vi "Main.vi"(10 "Game Settings":T1={"Control Device"=enum."Mouse", "Players Number"=4, "Score Limit"=3, "Difficulty"=1.0, "FPS"=8, "Mode"=enum."Solo"} {"FPS" items=["120"=8, "60"=16]; "Difficulty" items=["Hard"=1.0, "Medium"=0.8, "Easy"=0.6]; "Players Number" items=["2"=2, "4"=4]}) -> (0 "error out":errorcluster)   [LabVIEW 2021]
doc: "MIT Licence\nCopyright (c) 2024 David Grollier"
uses:
  Type Def/Game Settings.ctl
  Type Def/Control Device.ctl
  Type Def/Players Number.ctl
  Type Def/Difficulty.ctl
  Type Def/FPS.ctl
  Type Def/Mode.ctl
  Type Def/State Main.ctl
  Input Device/Keyboard/Keyboard.lvclass
  C:/Users/David/Documents/The-LabVIEW-Soccer-Game/Source/Input Device/Input Device.lvclass
  Input Device/Xbox Controller/Xbox Controller.lvclass
  Input Device/Mouse/Mouse.lvclass
  <vilib>/Platform/TimedLoop/XDataNode/timing_clust.ctl
  <vilib>/Platform/TimedLoop/XDataNode/nitl_modes.ctl
  <vilib>/Platform/TimedLoop/XDataNode/wakeup.ctl
  Game Componants/Game Componants.lvclass/Game Componants.ctl
  Input Device/Mouse/Mouse.lvclass/Mouse.ctl
  <extravilib>/ChannelInstances/Tag-a[.](class'Movable')/Read With Abort.vi
  <extravilib>/ChannelInstances/Tag-a[.](class'Movable')/Write With Abort.vi
  Game Componants/Game Board Component/Movable/Movable.lvclass
  C:/Users/David/Documents/The-LabVIEW-Soccer-Game/Source/Game Componants/Game Componants.lvclass
  <extravilib>/ChannelInstances/Tag-a[.](class'Movable')/Instantiate.vi
  <extravilib>/ChannelInstances/Tag-a[.](class'Movable')/EndpointRead.vi
  <extravilib>/ChannelInstances/Tag-a[.](class'Movable')/Endpoint.vi
  Input Device/Input Device.lvclass
  <vilib>/platform/TimedLoop/XDataNode/XDataNode.xnode
  AI Manager/AI Manager.lvclass
  Game Componants/Game Board/Game Board.lvclass
  <vilib>/Platform/TimedLoop/XDataNode/XDNodeRunTimeDep.lvlib
  Communication/Communication.lvclass
  Game Componants/Game Componants.lvclass
  <extravilib>/ChannelInstances/Tag-a[.](class'Movable').lvlib
panel:
  out "Display Action Info":string
  out "Display Direction Info":string
  out "Display info":string
  out "Score left":dbl
  out "Score right":dbl
  out "Game Board":picture
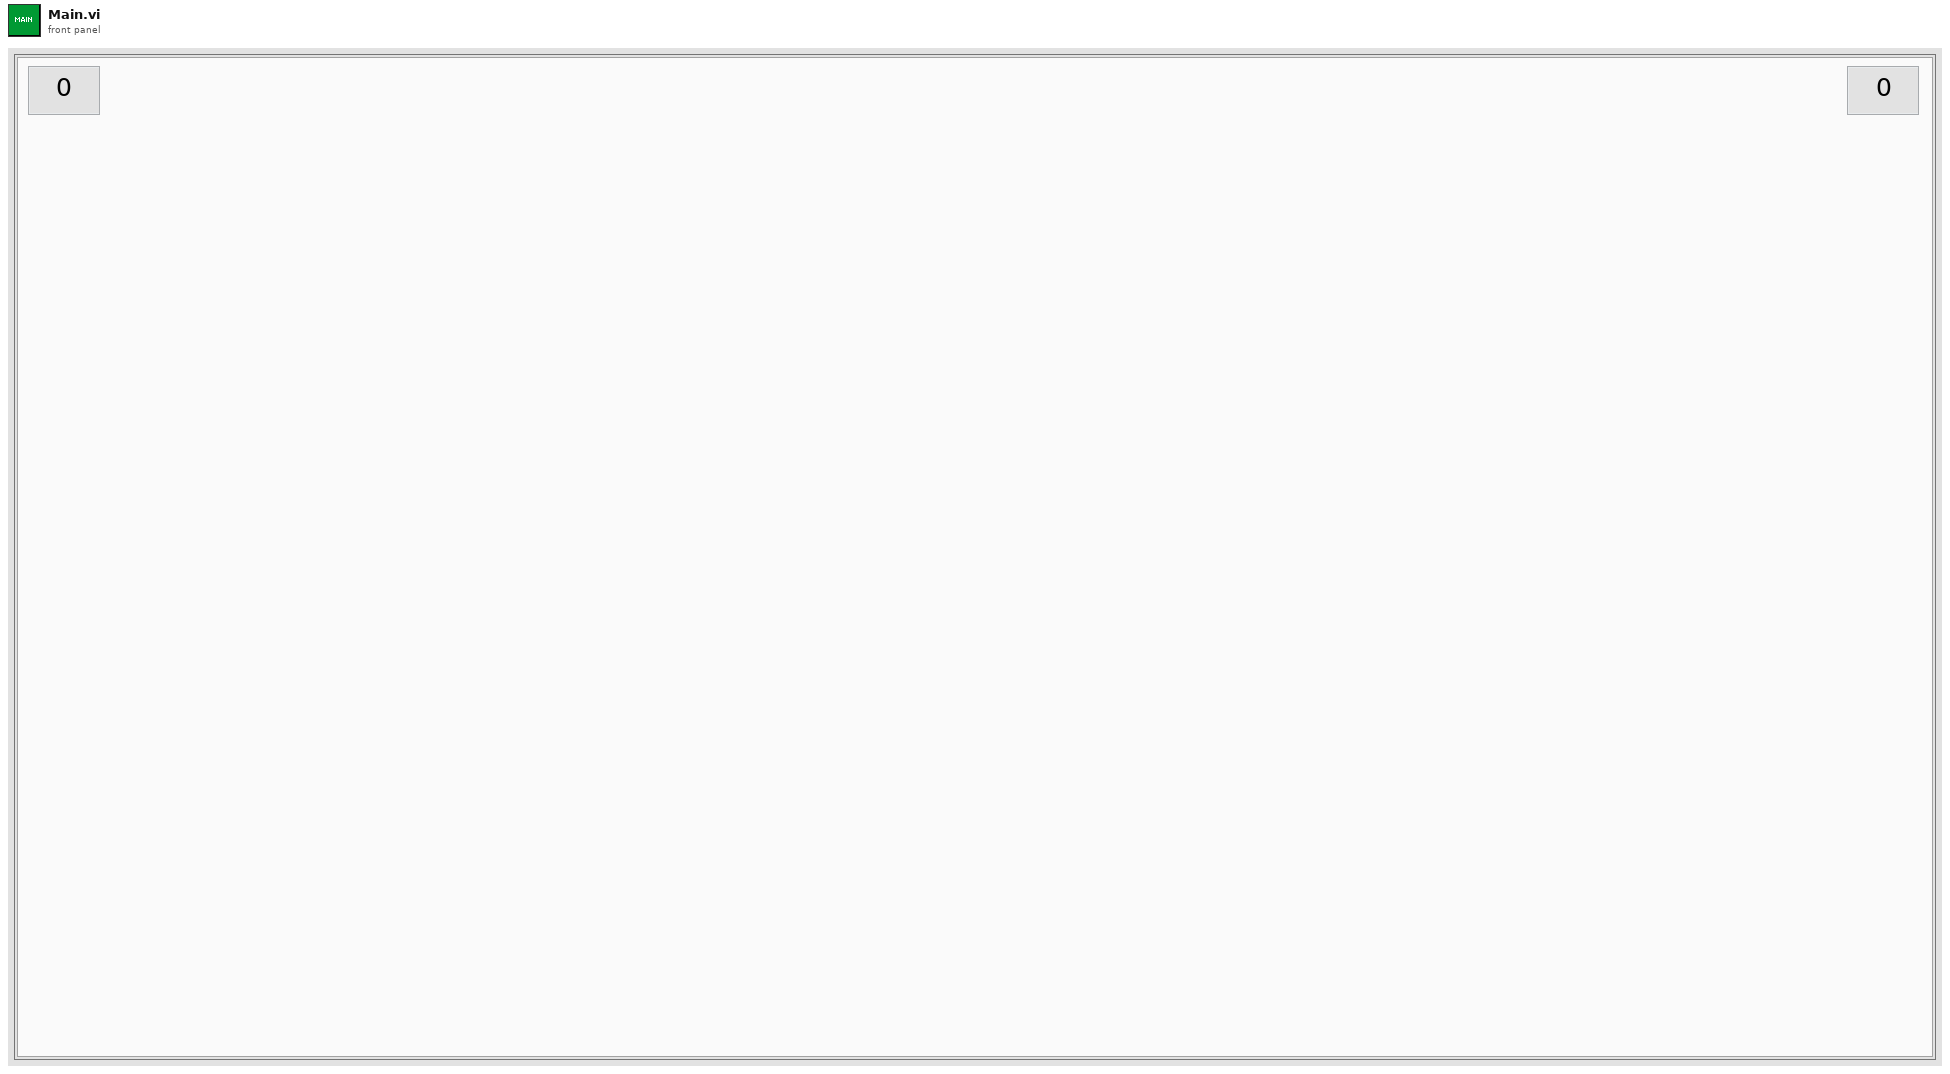
[diagram p1: front panel]
types:
  T1 = typedef "Game Settings.ctl" = cluster{"Control Device":T2, "Players Number":T3, "Score Limit":u8, "Difficulty":T4, "FPS":T5, "Mode":T6}
  T2 = typedef "Control Device.ctl" = enum16{"Arrow Keys", "Mouse", "Xbox Controller"}
  T3 = typedef "Players Number.ctl" = u16
  T4 = typedef "Difficulty.ctl" = dbl
  T5 = typedef "FPS.ctl" = u8
  T6 = typedef "Mode.ctl" = enum16{"Solo", "Multiplayer"}
  T7 = typedef "State Main.ctl" = enum16{"init", "Timer", "Playing"}
  T8 = typedef "XDNodeRunTimeDep.lvlib/timing_clust.ctl" = cluster{"Expected End [f-1]":u64, "Actual End [f-1]":u64, "Finished Late? [f-1]":bool, "Expected End [i-1]":u64, "Actual End [i-1]":u64, "Finished Late? [i-1]":bool, "Expected Start [i]":u64, "Actual Start [i]":u64, "Expected Start [f]":u64, "Actual Start [f]":u64, "Source Name":string, "Structure Name":string, "Period":i64, "Deadline":i64, "Offset":i64, "Start":i64, "Priority":i32, "Timeout":i32, "Mode":T9, "Wakeup Reason":T10, "Error":errorcluster, "Source Type":string, "Secondary Source Type":string, "Global End Time":u64, "Global Start Time":u64, "Frame Duration":u64, "Iteration Duration":u64, "Assigned CPU":i32, "I/O Scan Engine Mode":u32}
  T9 = typedef "XDNodeRunTimeDep.lvlib/nitl_modes.ctl" = enum32{"No Change", "Process missed periods, maintain original phase", "Discard missed periods, maintain original phase", "Process missed periods, ignore original phase", "Discard missed periods, ignore original phase"}
  T10 = typedef "XDNodeRunTimeDep.lvlib/wakeup.ctl" = enum32{"Normal", "Aborted", "Asynchronous wakeup", "Timing source error", "Timed loop error", "Timeout"}
  T11 = typedef "Tag-a[.](class'Movable').lvlib/))Channel.ctl" = refnum<queue>
  T12 = typedef "LVBoundsTypeDef.ctl" = cluster{"Width":u32, "Height":u32}
  T13 = typedef "Coordinates.ctl" = cluster{"x":dbl, "y":dbl}
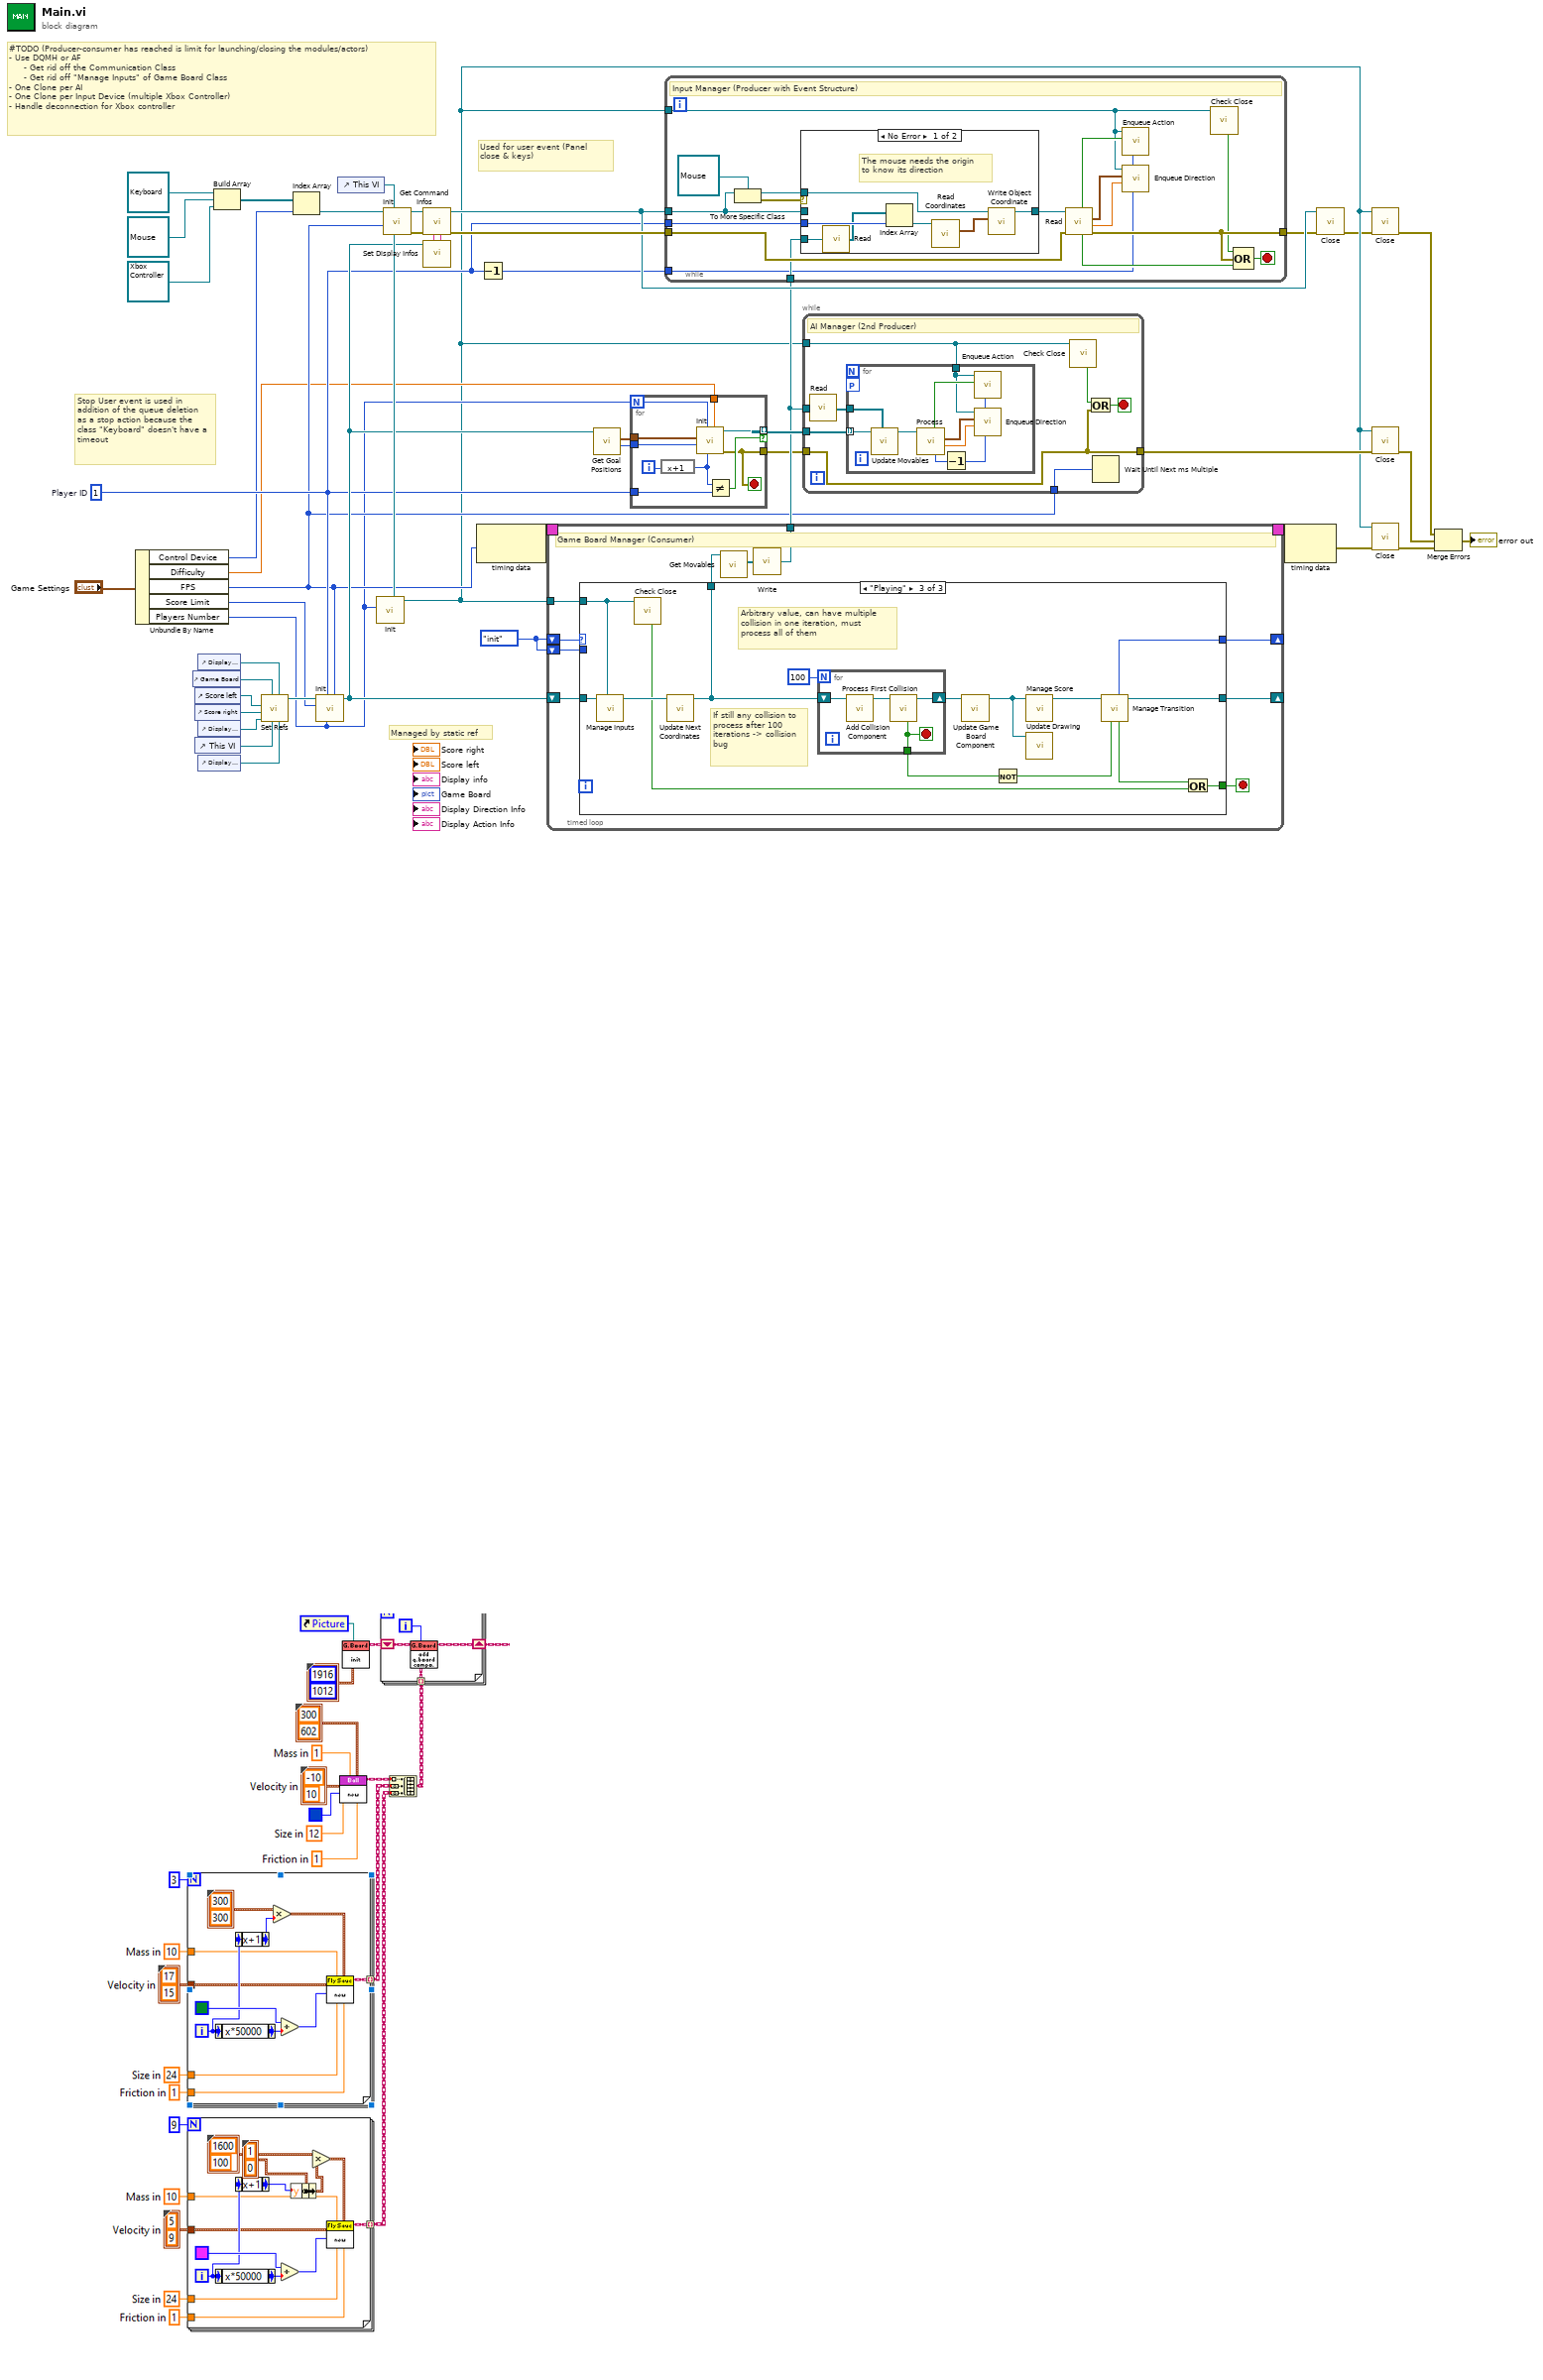
[diagram p0: block diagram]
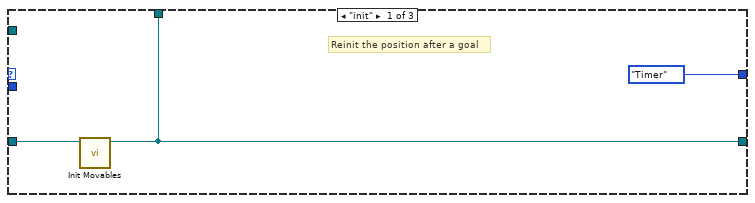
[diagram p3: hidden frame]
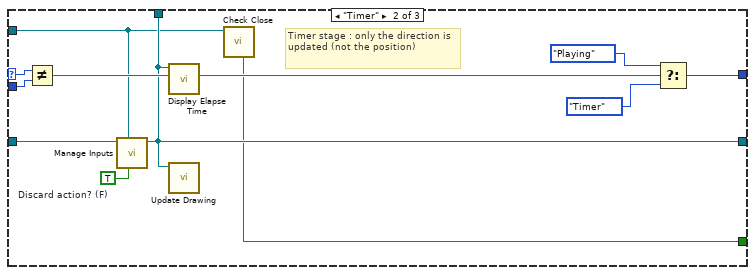
[diagram p4: hidden frame]
diagram:
  w21 = i64 1  # Player ID
  w44 = State_Main."init"
  # "Used for user event (Panel close & keys)"
  # "Stop User event is used in addition of the queue deletion as a stop action because the class \"Keyboard\" doesn't have a timeout"
  # "#TODO (Producer-consumer has reached is limit for launching/closing the modules/actors)\n- Use DQMH or AF  \n     - Get rid off the Communication Class\n     - Get rid off \"Manage Inputs\" of Game Board Class \n- One Clone per AI\n- One Clone per Input Device (multiple Xbox Controller)\n- Handle deconnection for Xbox controller"
  # "Managed by static ref"
  n1 = Unbundle By Name("Game Settings") -> ("Control Device"=w13:T2, "Difficulty"=w5:T4, "FPS"=w12:T5, "Score Limit"=w11:u8, "Players Number"=w10:T3)
  n2 = control-ref of="Game Board"() -> (w42:refnum<vi>)
  n3 = control-ref of="Score left"() -> (w40:refnum<vi>)
  n4 = control-ref of="Score right"() -> (w41:refnum<vi>)
  n5 = control-ref of="This VI"() -> (w37:refnum<vi>)
  n6 = control-ref of="Display Action Info"() -> (w23:refnum<vi>)
  n7 = control-ref of="Display info"() -> (w38:refnum<vi>)
  n8 = control-ref of="Display info help"() -> (w33:refnum<vi>)
  n9 = Build Array(refnum<class "Keyboard.lvclass"> refnum ("Keyboard.lvclass"), refnum<class "Mouse.lvclass"> refnum ("Mouse.lvclass"), refnum<class "Xbox Controller.lvclass"> refnum ("Xbox Controller.lvclass")) -> (w16:refnum<class "Input Device.lvclass">[])
  n10 = call "Set Refs.vi"("Display Direction in"=w33, "Display Action Info in"=w23, "VI ref in"=w37, "Game Board ref in"=w42, "Display info in"=w38, "Score right in"=w41, "Score left in"=w40) -> ("Game Board out"=w39:refnum<class "Game Board.lvclass">)  [unwired: 4 in]
  n11 = Index Array(array=w16, index=w13) -> (element=w15:refnum<class "Input Device.lvclass">)
  n12 = call "Init.vi"("Period (ms) in"=w12, "Players number in"=w10, "Player ID in"=w21, "Score to win in"=w11, "Game Board in"=w39) -> ("Game Board out"=w22:refnum<class "Game Board.lvclass">)  [unwired: 6 in]
  n13 = control-ref of="This VI"() -> (w31:refnum<vi>)
  n14 = call "Init.vi"("Players number in"=w10) -> ("Communication out"=w2:refnum<class "Communication.lvclass">, "Stop User Event out"=w30:refnum<user-event>)  [unwired: 9 in]
  n15 = call-dynamic "Init.vi"("Stop User Event in"=w30, "Ref FP in"=w31, "Period (ms) in"=w12, "Input Device in"=w15) -> ("error out"=w32:errorcluster, "Input Device out"=w27:refnum<class "Input Device.lvclass">)  [unwired: 6 in]
  n16 = call-dynamic "Get Command Infos.vi"("error in (no error)"=w32, "Input Device in"=w27) -> ("error out"=w28:errorcluster, "Input Device out"=w26:refnum<class "Input Device.lvclass">, "Direction info out"=w24:string, "Boost info out"=w25:string)  [unwired: 6 in]
  n17 = call "Set Display Infos.vi"("Direction info in"=w24, "Boost info in"=w25, "Game Board in"=w22) -> ()  [unwired: 9 in]
  n18 = node-c288(w12) -> (w47:T8)
  n19 = Decrement(x=w21) -> (x-1=w3:i64)
  n20 = timed-loop {
    tunnel: w2 -> [w52]
    shift-right: [w56] -> _
    shift-left: w22 -> [w57]
    timing: w47 -> [_]
    timing-out: [_] -> w46
    shift-right: [w53] -> _
    shift-left: w44 -> [w54]
    shift-left: w44 -> [w51]
    tunnel: [w48] -> w20
    stop <- w55 stop-if-true
    # "Game Board Manager (Consumer)"
    n21 = case shown="\"Playing\"" w54 {
      selector: w54 -> [_ w70 _]
      tunnel: w57 -> [w59 w65 w76]
      tunnel: [w58 w63 w80] -> w56
      tunnel: [_ w61 w77] -> w55
      tunnel: w52 -> [_ w62 w74]
      tunnel: [State_Main."Timer" w71 w79] -> w53
      tunnel: w51 -> [_ w69 _]
      tunnel: [w58 w63 w75] -> w50
      frame "init" {
        # "Reinit the position after a goal"
        n22 = call "Init Movables.vi"("Game Board in"=w59) -> ("Game Board out"=w58:refnum<class "Game Board.lvclass">)  [unwired: 10 in]
      }
      frame "Timer" {
        w64 = TRUE  # Discard action? (F)
        # "Timer stage : only the direction is updated (not the position)"
        # "State timer, only the direction is updated (not the position)"
        n23 = Not Equal?(x=w70, y=w69) -> (x != y?=w68:bool)
        n24 = call "Manage Inputs.vi"("Discard action? (F)"=w64, "Communication in"=w62, "Game Board in"=w65) -> ("Game Board out"=w63:refnum<class "Game Board.lvclass">)  [unwired: 8 in]
        n25 = call "Display Elapse Time.vi"("Reset?"=w68, "Game Board in"=w63) -> ("Time has Elapsed?"=w67:bool)  [unwired: 9 in]
        n26 = call "Update Drawing.vi"("Game Board in"=w63) -> ()  [unwired: 11 in]
        n27 = call "Check Close.vi"("Communication in"=w62) -> ("Stop?"=w61:bool)  [unwired: 10 in]
        n28 = Select(t=State_Main."Playing", s=w67, f=State_Main."Timer") -> (s? t:f=w71:T7)
      }
      frame "Playing" {
        # "If still any collision to process after 100 iterations -> collision bug"
        # "Arbitrary value, can have multiple collision in one iteration, must process all of them"
        # "Game engine"
        n29 = call "Manage Inputs.vi"("Communication in"=w74, "Game Board in"=w76) -> ("Game Board out"=w84:refnum<class "Game Board.lvclass">)  [unwired: 9 in]
        n30 = call "Check Close.vi"("Communication in"=w74) -> ("Stop?"=w73:bool)  [unwired: 10 in]
        n31 = call "Update Next Coordinates.vi"("Game Board in"=w84) -> ("Game Board out"=w75:refnum<class "Game Board.lvclass">)  [unwired: 10 in]
        n32 = for {
          N: 100 -> [_]
          shift-right: [w90] -> w86
          shift-left: w75 -> [w89]
          tunnel: [w88] -> w87
          stop <- w88 stop-if-true
          n33 = call "Add Collision Component .vi"("Game Board in"=w89) -> ("Game Board out"=w91:refnum<class "Game Board.lvclass">)  [unwired: 10 in]
          n34 = call "Process First Collision.vi"("Game Board in"=w91) -> ("Game Board out"=w90:refnum<class "Game Board.lvclass">, "empty collision?"=w88:bool)  [unwired: 9 in]
        }
        n35 = call "Update Game Board Component.vi"("Game Board in"=w86) -> ("Game Board out"=w83:refnum<class "Game Board.lvclass">)  [unwired: 10 in]
        n36 = Not(x=w87) -> (.not. x?=w81:bool)
        n37 = call "Manage Score.vi"("Game Board in"=w83) -> ("Game Board out"=w82:refnum<class "Game Board.lvclass">)  [unwired: 10 in]
        n38 = call "Update Drawing.vi"("Game Board in"=w83) -> ()  [unwired: 11 in]
        n39 = call "Manage Transition.vi"("Force transition"=w81, "Game Board in"=w82) -> ("Game Board out"=w80:refnum<class "Game Board.lvclass">, "Exit?"=w78:bool, "State out"=w79:T7)  [unwired: 7 in]
        n40 = Or(x=w78, y=w73) -> (x .or. y?=w77:bool)
      }
    }
    n41 = call "Get Movables.vi"("Game Board in"=w50) -> ("Movables out"=w49:refnum<class "Movable.lvclass">[])  [unwired: 10 in]
    n42 = call <extravilib>:"Write.vi"("element"=w49) -> ("channel"=w48:T11)  [unwired: 1 out]
  }
  n43 = call "Get Goal Positions.vi"("Game Board in"=w22) -> ("Width goal out"=w35:u16, "Bounds out"=w36:T12)  [unwired: 9 in]
  n44 = for {
    N: w10 -> [w96]
    tunnel: [w103] -> w34 mode=indexing if=w97
    tunnel: w35 -> [w102]
    tunnel: w36 -> [w101]
    tunnel: w21 -> [w98]
    tunnel: w5 -> [w95]
    tunnel: [w94] -> w9
    i -> [w100]
    stop <- w94 stop-if-true
    n45 = expression code="x+1"(w100) -> (w99:i32)
    n46 = call "Init.vi"("Difficulty"=w95, "Self Index in"=w99, "Players number in"=w96, "Right width goal in"=w102, "Bounds in"=w101) -> ("error out"=w94:errorcluster, "AI Manager out"=w103:refnum<class "AI Manager.lvclass">)  [unwired: 5 in]
    n47 = Not Equal?(x=w99, y=w98) -> (x != y?=w97:bool)
  }
  n48 = while {
    tunnel: w28 -> [w112]
    tunnel: w26 -> [w115]
    tunnel: [w120] -> w4
    tunnel: w21 -> [w111]
    tunnel: w20 -> [w110]
    tunnel: w2 -> [w108]
    tunnel: w3 -> [w104]
    stop <- w118 stop-if-true
    # "Input Manager (Producer with Event Structure)"
    n49 = To More Specific Class(target class=refnum<class "Mouse.lvclass"> refnum ("Mouse.lvclass"), reference=w115) -> (specific class reference=w113:refnum<class "Mouse.lvclass">, error out=w116:errorcluster)  [unwired: 1 in]
    n50 = case shown="No Error" w116 {
      tunnel: w115 -> [_ w128]
      tunnel: [w126 w128] -> w114
      tunnel: w113 -> [w127 _]
      tunnel: w111 -> [w125 _]
      tunnel: w110 -> [w122 _]
      frame No Error {
        # "The mouse needs the origin to know its direction"
        n51 = call <extravilib>:"Read.vi"("channel"=w122) -> ("element"=w121:refnum<class "Movable.lvclass">[])  [unwired: 1 in, 1 out]
        n52 = Index Array(array=w121, index=w125) -> (element=w124:refnum<class "Movable.lvclass">)
        n53 = call "Read Coordinates.vi"("Game Componants in"=w124) -> ("Coordinates"=w123:T13)  [unwired: 10 in]
        n54 = call "Write Object Coordinate.vi"("Object Coordinate"=w123, "Mouse in"=w127) -> ("Mouse out"=w126:refnum<class "Mouse.lvclass">)  [unwired: 9 in]
      }
      frame Error {
      }
    }
    n55 = call-dynamic <extravilib>:"Read.vi"("error in (no error)"=w112, "Input Device in"=w114) -> ("error out"=w120:errorcluster, "Velocity out"=w106:dbl, "Direction out"=w107:cluster{dbl, dbl}, "Stop?"=w119:bool, "Boost?"=w109:bool)  [unwired: 5 in]
    n56 = call "Enqueue Action.vi"("Index in"=w104, "Boost in"=w109, "Communication in"=w108) -> ()  [unwired: 9 in]
    n57 = call "Enqueue Direction.vi"("Index in"=w104, "Velocity in"=w106, "Direction in"=w107, "Communication in"=w108) -> ()  [unwired: 8 in]
    n58 = call "Check Close.vi"("Communication in"=w108) -> ("Stop?"=w105:bool)  [unwired: 10 in]
    n59 = Compound Arithmetic op=OR(w105, w120, w119) -> (w118:bool)
  }
  n60 = while {
    tunnel: w2 -> [w129]
    tunnel: w34 -> [w136]
    tunnel: w12 -> [w135]
    tunnel: w20 -> [w134]
    tunnel: w9 -> [w130]
    tunnel: [w130] -> w8
    stop <- w131 stop-if-true
    # "AI Manager (2nd Producer)"
    n61 = call <extravilib>:"Read.vi"("channel"=w134) -> ("element"=w133:refnum<class "Movable.lvclass">[])  [unwired: 1 in, 1 out]
    n62 = for {
      tunnel: w136 -> [w145] mode=indexing
      tunnel: w133 -> [w143]
      workers-P: _ -> [_]
      tunnel: w129 -> [w140]
      n63 = call "Update Movables.vi"("Movables in"=w143, "AI Manager in"=w145) -> ("AI Manager out"=w144:refnum<class "AI Manager.lvclass">)  [unwired: 9 in]
      n64 = call "Process.vi"("AI Manager in"=w144) -> ("Velocity out"=w139:dbl, "Direction out"=w141:cluster{dbl, dbl}, "Self Index out"=w138:i32, "Boost ?"=w142:bool)  [unwired: 7 in]
      n65 = Decrement(x=w138) -> (x-1=w137:i32)
      n66 = call "Enqueue Action.vi"("Index in"=w137, "Boost in"=w142, "Communication in"=w140) -> ()  [unwired: 9 in]
      n67 = call "Enqueue Direction.vi"("Index in"=w137, "Velocity in"=w139, "Direction in"=w141, "Communication in"=w140) -> ()  [unwired: 8 in]
    }
    n68 = call "Check Close.vi"("Communication in"=w129) -> ("Stop?"=w132:bool)  [unwired: 10 in]
    n69 = Or(x=w132, y=w130) -> (x .or. y?=w131:bool)
    n70 = Wait Until Next ms Multiple(millisecond multiple=w135) -> ()  [unwired: 1 out]
  }
  n71 = node-c288(w46) -> (w29:errorcluster)
  n72 = call-dynamic "Close.vi"("error in (no error)"=w4, "Input Device in"=w26) -> ("error out"=w1:errorcluster)  [unwired: 9 in]
  n73 = call "Close.vi"("error in (no error)"=w1, "Communication in"=w2) -> ("error out"=w6:errorcluster)  [unwired: 9 in]
  n74 = call "Close.vi"("error in (no error)"=w8, "Communication in"=w2) -> ("error out"=w7:errorcluster)  [unwired: 9 in]
  n75 = call "Close.vi"("error in (no error)"=w29, "Communication in"=w2) -> ("error out"=w45:errorcluster)  [unwired: 9 in]
  n76 = Merge Errors(w6, w7, w45) -> (→"error out":errorcluster)
